vi "animation.vi"() -> ()   [LabVIEW 2015]
panel:
  in  "stop":bool
  out "Pict Ring":u16(ring)
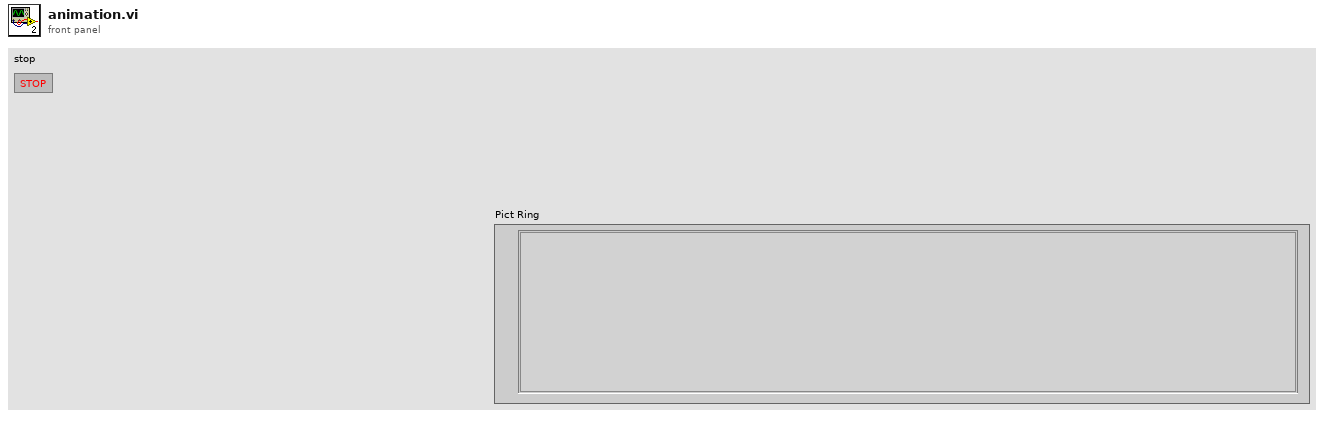
[diagram p1: front panel]
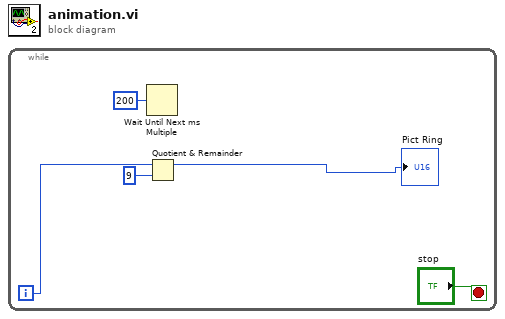
[diagram p0: block diagram]
diagram:
  n1 = while {
    i -> [w5]
    stop <- "stop" stop-if-true
    n2 = Wait Until Next ms Multiple(millisecond multiple=u32 200) -> ()  [unwired: 1 out]
    n3 = Quotient & Remainder(x=w5, y=9) -> (x-y*floor(x/y)=→"Pict Ring":i32)  [unwired: 1 out]
  }
